vi "OR16x16.vi"(1 "B":bool[][](array[boolean])=[[FALSE, FALSE, FALSE, FALSE], [FALSE, FALSE, FALSE, FALSE], [FALSE, FALSE, FALSE, FALSE], [FALSE, FALSE, FALSE, FALSE]], 2 "A":bool[][](array[boolean])=[[FALSE, FALSE, FALSE, FALSE], [FALSE, FALSE, FALSE, FALSE], [FALSE, FALSE, FALSE, FALSE], [FALSE, FALSE, FALSE, FALSE]]) -> (0 "z":bool[][](array[boolean]))   [LabVIEW 2012]
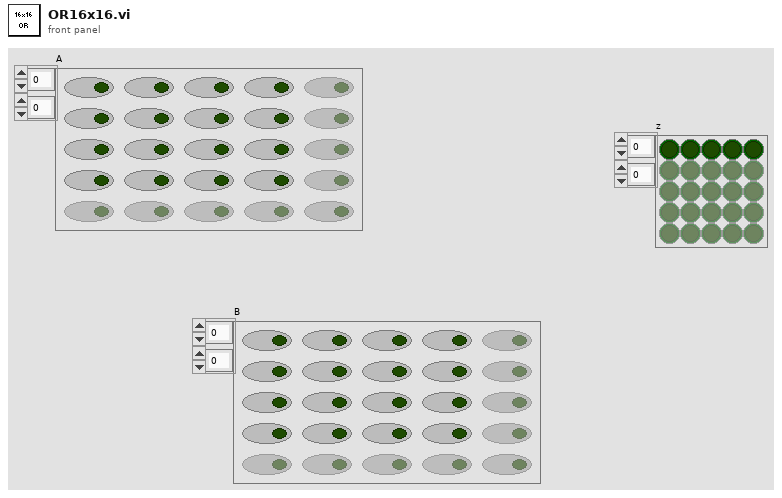
[diagram p1: front panel]
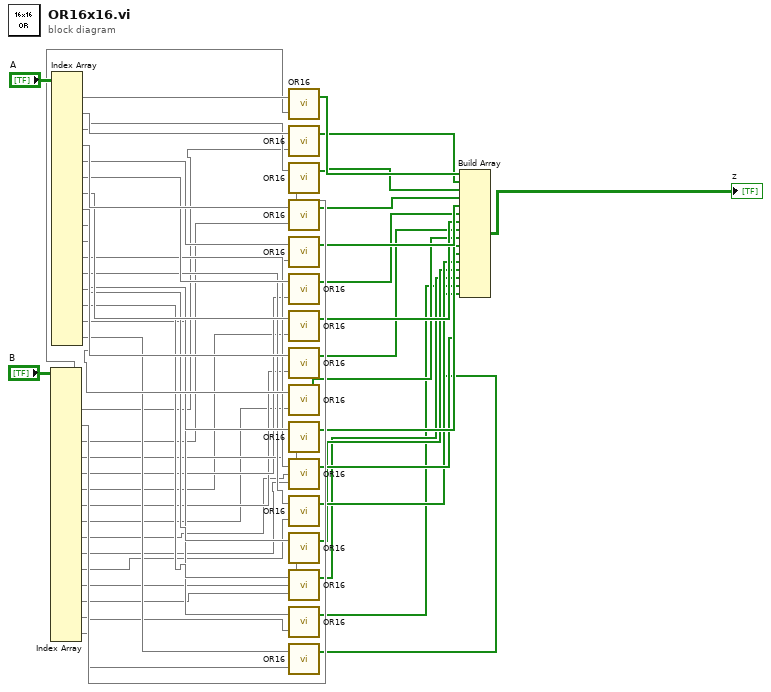
[diagram p0: block diagram]
diagram:
  n1 = Index Array(array="B") -> (element #1=w33:bool[], element #2=w32:bool[], element #3=w31:bool[], element #4=w30:bool[], element #5=w29:bool[], element #6=w28:bool[], element #7=w27:bool[], element #8=w26:bool[], element #9=w25:bool[], element #10=w24:bool[], element #11=w23:bool[], element #12=w22:bool[], element #13=w21:bool[], element #14=w20:bool[], element #15=w19:bool[], element #16=w18:bool[])  [unwired: 32 in]
  n2 = Index Array(array="A") -> (element #1=w49:bool[], element #2=w48:bool[], element #3=w47:bool[], element #4=w46:bool[], element #5=w45:bool[], element #6=w44:bool[], element #7=w43:bool[], element #8=w42:bool[], element #9=w41:bool[], element #10=w40:bool[], element #11=w39:bool[], element #12=w38:bool[], element #13=w37:bool[], element #14=w36:bool[], element #15=w35:bool[], element #16=w34:bool[])  [unwired: 32 in]
  n3 = call "OR16.vi"("B"=w33, "A"=w49) -> ("z"=w17:bool[])  [unwired: 1 out]
  n4 = call "OR16.vi"("B"=w32, "A"=w48) -> ("z"=w16:bool[])  [unwired: 1 out]
  n5 = call "OR16.vi"("B"=w31, "A"=w47) -> ("z"=w15:bool[])  [unwired: 1 out]
  n6 = call "OR16.vi"("B"=w30, "A"=w46) -> ("z"=w14:bool[])  [unwired: 1 out]
  n7 = call "OR16.vi"("B"=w29, "A"=w45) -> ("z"=w13:bool[])  [unwired: 1 out]
  n8 = call "OR16.vi"("B"=w28, "A"=w44) -> ("z"=w12:bool[])  [unwired: 1 out]
  n9 = call "OR16.vi"("B"=w27, "A"=w43) -> ("z"=w11:bool[])  [unwired: 1 out]
  n10 = call "OR16.vi"("B"=w26, "A"=w42) -> ("z"=w10:bool[])  [unwired: 1 out]
  n11 = call "OR16.vi"("B"=w25, "A"=w41) -> ("z"=w9:bool[])  [unwired: 1 out]
  n12 = call "OR16.vi"("B"=w24, "A"=w40) -> ("z"=w8:bool[])  [unwired: 1 out]
  n13 = call "OR16.vi"("B"=w23, "A"=w39) -> ("z"=w7:bool[])  [unwired: 1 out]
  n14 = call "OR16.vi"("B"=w22, "A"=w38) -> ("z"=w6:bool[])  [unwired: 1 out]
  n15 = call "OR16.vi"("B"=w21, "A"=w37) -> ("z"=w5:bool[])  [unwired: 1 out]
  n16 = call "OR16.vi"("B"=w20, "A"=w36) -> ("z"=w4:bool[])  [unwired: 1 out]
  n17 = call "OR16.vi"("B"=w19, "A"=w35) -> ("z"=w3:bool[])  [unwired: 1 out]
  n18 = call "OR16.vi"("B"=w18, "A"=w34) -> ("z"=w2:bool[])  [unwired: 1 out]
  n19 = Build Array(w17, w16, w15, w14, w13, w12, w11, w10, w9, w8, w7, w6, w5, w4, w3, w2) -> (→"z":bool[][])
